vi "Get Full Decay Fit & Residual Plots (1-Exp Fit).vi"(4 "Laser Period":dbl[unit], 6 "Fit Options":T2={"Show Fit Residuals"=TRUE, "Fit Model"=enum."1-Exponential", "Residual Type"=enum."Standard", "Max Decay Percentile"=0.0, "Min Decay Percentile"=0.0, "Show Full Decay"=TRUE, "Weights"=enum."Unweighted", "Fitting Method"=enum."Least Square", "Compute Parameter Uncertainties"=TRUE, "Periodic Boundaries"=TRUE, "Model Calculation"=enum."Simulation", "Period"=1.2500000000000001e-08, "Termination Criteria"={"Max Iterations"=1000, "Max Function Calls"=0, "Max Time"=1000.0, "Function Tolerance"=1e-06, "Parameter Tolerance"=1e-06, "Gradient Tolerance"=0.0, "Min Lambda"=1e-06, "Max Lambda"=1e-06, "Initial Tick Count"=0}, "Offset Resolution"=1.2500000000000001e-08, "Use Local IRF"=TRUE, "Fitting Algorithm"=enum."Levenberg-Marquardt", "Show Confidence Interval "=TRUE, "Confidence Level"=95.0} {"Confidence Level" min=0.0 max=100.0; "Offset Resolution" min=0.0; "Period" min=0.0; "Min Decay Percentile" min=0.0 max=1.0; "Max Decay Percentile" min=0.0 max=100.0}, 8 "Error In":errorcluster, 9 "Best Fit Parameters (All)":dbl[](array[numeric]), 10 "IRF":cluster{"t Array":dbl[], "IRF Array":dbl[]}, 11 "Full Decay":cluster{"t Array":dbl[], "Y Array":dbl[]}) -> (0 "Error Out":errorcluster, 3 "Fit Plots":T1)   [LabVIEW 2021, in "Fits.lvlib"]
uses:
  Fits.lvlib
  Decay Fit Options v4.ctl
  Decay Convolution/Decay Model.ctl
  Residual Type.ctl
  Fit Weights Type v2.ctl
  Non-linear Fitting Method v2.ctl
  Fit Calculation Method.ctl
  Non-linear Fitting Algorithm.ctl
  Fit Plots.ctl
  Decay Convolution/Fit Control Data.ctl
  Graphs/XY Graph/XY Graph Plot Data.ctl
  Graphs/XY Graph/XY Graph Add-Ons.lvlib
panel:
  out "XY Graph":cluster{"t Array":dbl[], "f(X,a)":dbl[]}[](graph)
  # "see the License on the block diagram (Ctrl+E or Window:Show Block Diagram)"
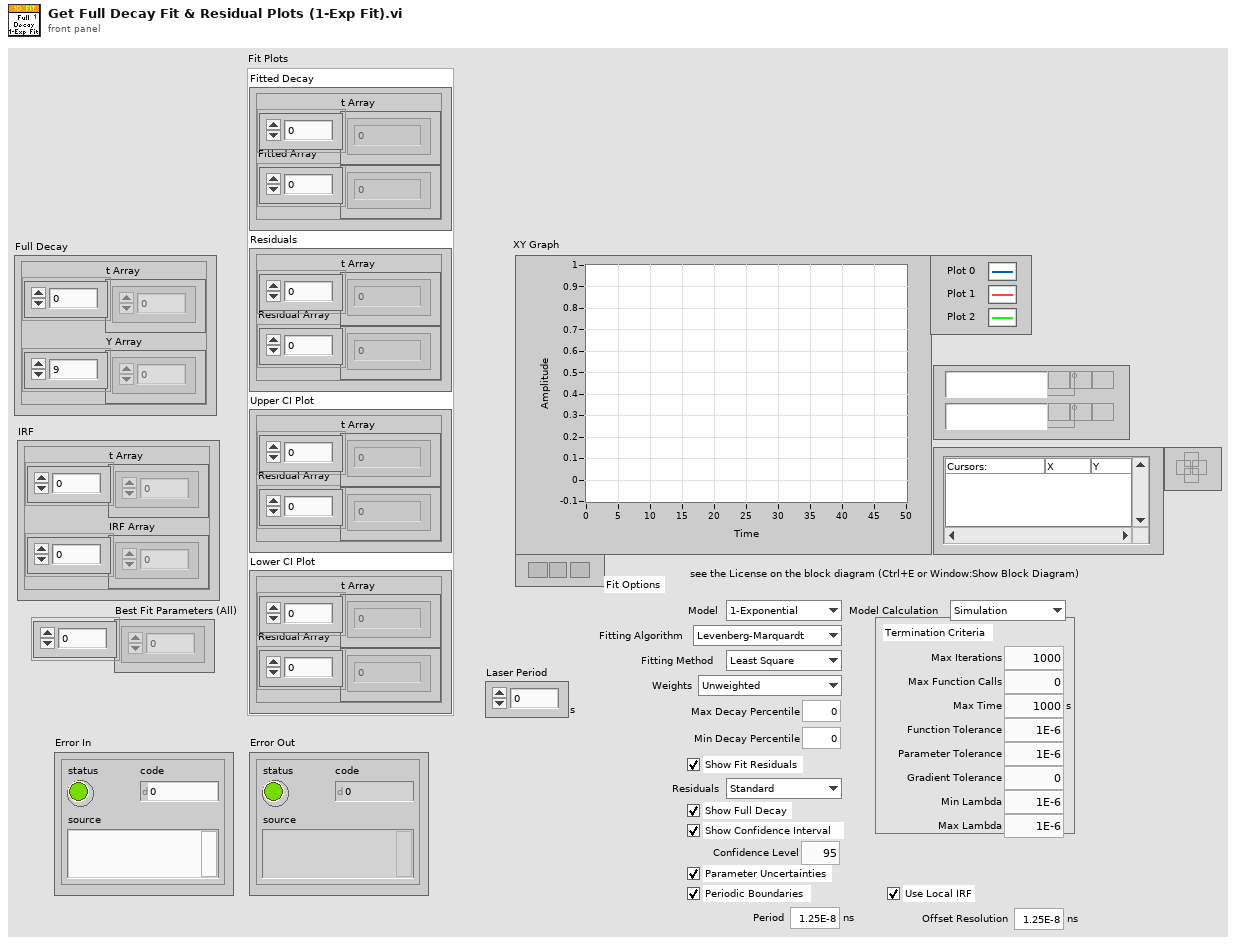
[diagram p1: front panel]
types:
  T1 = typedef "Fits.lvlib/Fit Plots.ctl" = cluster{"Fitted Decay":cluster{"t Array":dbl[], "Fitted Array":dbl[]}, "Residuals":cluster{"t Array":dbl[], "Residual Array":dbl[]}, "Upper CI Plot":cluster{"t Array":dbl[], "Residual Array":dbl[]}, "Lower CI Plot":cluster{"t Array":dbl[], "Residual Array":dbl[]}}
  T2 = typedef "Fits.lvlib/Decay Fit Options v4.ctl" = cluster{"Show Fit Residuals":bool, "Fit Model":T3, "Residual Type":T4, "Max Decay Percentile":dbl, "Min Decay Percentile":dbl, "Show Full Decay":bool, "Weights":T5, "Fitting Method":T6, "Compute Parameter Uncertainties":bool, "Periodic Boundaries":bool, "Model Calculation":T7, "Period":dbl[unit], "Termination Criteria":cluster{"Max Iterations":i32, "Max Function Calls":i32, "Max Time":dbl[unit], "Function Tolerance":dbl, "Parameter Tolerance":dbl, "Gradient Tolerance":dbl, "Min Lambda":dbl, "Max Lambda":dbl, "Initial Tick Count":u32}, "Offset Resolution":dbl[unit], "Use Local IRF":bool, "Fitting Algorithm":T8, "Show Confidence Interval ":bool, "Confidence Level":dbl}
  T3 = typedef "Fits.lvlib/Decay Model.ctl" = enum16{"1-Exponential", "2-Exponentials"}
  T4 = typedef "Fits.lvlib/Residual Type.ctl" = enum16{"Standard", "Normalized", "Reduced"}
  T5 = typedef "Fits.lvlib/Fit Weights Type v2.ctl" = enum16{"Unweighted", "1/Variance (Neyman)", "1/Variance (Pearson)", "Best of All"}
  T6 = typedef "Fits.lvlib/Non-linear Fitting Method v2.ctl" = enum16{"Least Square", "Least Absolute Residual", "Bisquare", "MLE", "-", "Best of All"}
  T7 = typedef "Fits.lvlib/Fit Calculation Method.ctl" = enum16{"Simulation", "Convolution", "Integration"}
  T8 = typedef "Fits.lvlib/Non-linear Fitting Algorithm.ctl" = enum16{"Levenberg-Marquardt", "Trust-Region Dogleg"}
  T9 = typedef "Fits.lvlib/Fit Control Data.ctl" = cluster{"IRF":T10, "Laser Period":dbl, "SYNC Period":dbl}
  T10 = typedef "XY Graph Add-Ons.lvlib/XY Graph Plot Data.ctl" = cluster{"X Array":dbl[], "Y Array":dbl[]}
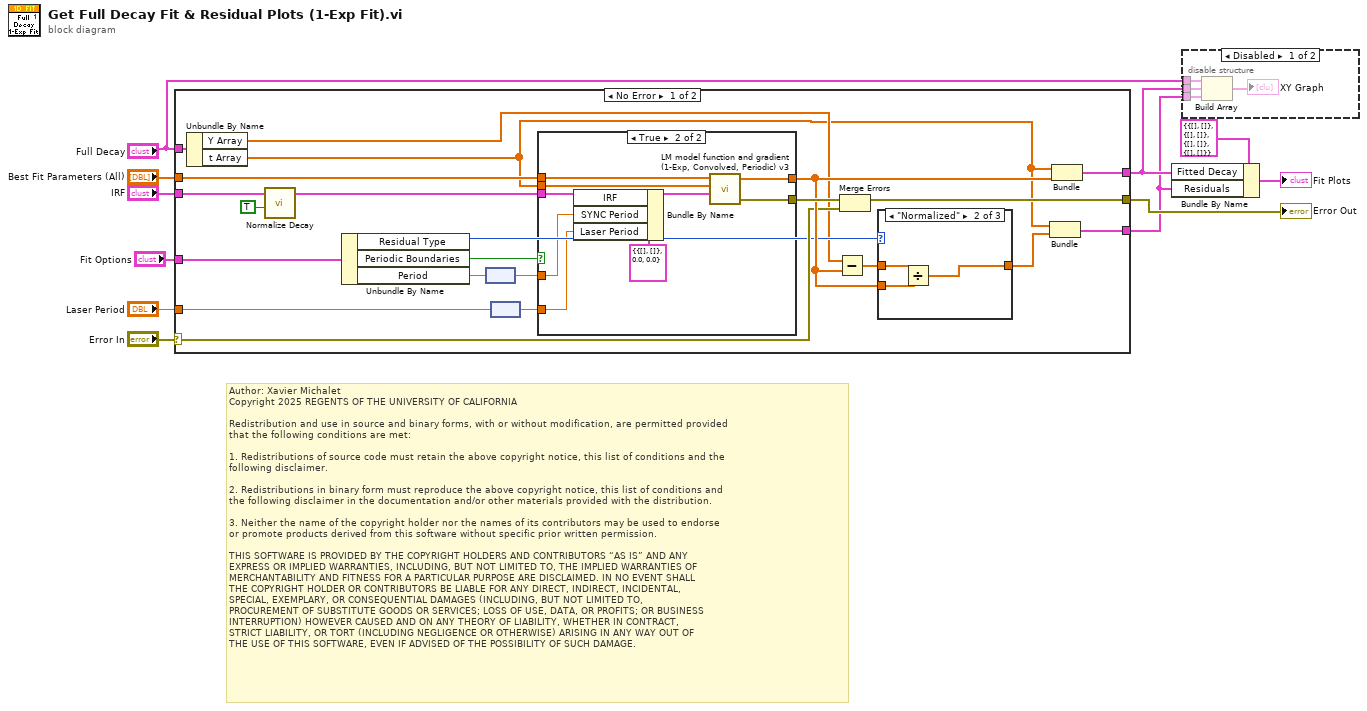
[diagram p0: block diagram]
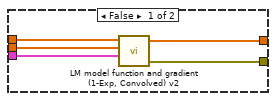
[diagram p3: hidden frame]
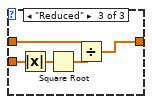
[diagram p5: hidden frame]
diagram:
  # "Author: Xavier Michalet\nCopyright 2025 REGENTS OF THE UNIVERSITY OF CALIFORNIA\n\nRedistribution and use in source and binary forms, with or without modification, are permitted provided\nthat the following conditions are met:\n\n1. Redistributions of source code must retain the above copyright notice, this list of conditions and the\nfollowing disclaimer.\n\n2. Redistributions in binary form must reproduce the above copyright notice, this list of conditions and\nthe following disclaimer in the documentation and/or other materials provided with the distribution.\n\n3. Neither the name of the copyright holder nor the names of its contributors may be used to endorse \nor promote products derived from this software without specific prior written permission.\n\nTHIS SOFTWARE IS PROVIDED BY THE COPYRIGHT HOLDERS AND CONTRIBUTORS “AS IS” AND ANY \nEXPRESS OR IMPLIED WARRANTIES, INCLUDING, BUT NOT LIMITED TO, THE IMPLIED WARRANTIES OF\nMERCHANTABILITY AND FITNESS FOR A PARTICULAR PURPOSE ARE DISCLAIMED. IN NO EVENT SHALL\nTHE COPYRIGHT HOLDER OR CONTRIBUTORS BE LIABLE FOR ANY DIRECT, INDIRECT, INCIDENTAL, \nSPECIAL, EXEMPLARY, OR CONSEQUENTIAL DAMAGES (INCLUDING, BUT NOT LIMITED TO, \nPROCUREMENT OF SUBSTITUTE GOODS OR SERVICES; LOSS OF USE, DATA, OR PROFITS; OR BUSINESS\nINTERRUPTION) HOWEVER CAUSED AND ON ANY THEORY OF LIABILITY, WHETHER IN CONTRACT, \nSTRICT LIABILITY, OR TORT (INCLUDING NEGLIGENCE OR OTHERWISE) ARISING IN ANY WAY OUT OF\nTHE USE OF THIS SOFTWARE, EVEN IF ADVISED OF THE POSSIBILITY OF SUCH DAMAGE."
  n1 = case shown="No Error" "Error In" {
    selector: "Error In" -> [w23 w57]
    tunnel: "IRF" -> [w16 _]
    tunnel: "Best Fit Parameters (All)" -> [w25 _]
    tunnel: [w33 _] -> w2
    tunnel: "Fit Options" -> [w32 _]
    tunnel: [w24 w57] -> w8
    tunnel: [w29 _] -> w1
    tunnel: "Full Decay" -> [w27 _]
    tunnel: "Laser Period" -> [w22 _]
    frame No Error {
      n2 = Unbundle By Name(w27) -> ("Y Array"=w13:dbl[], "t Array"=w12:dbl[])
      n3 = call "Normalize Decay.vi"("IRF (F)"=TRUE, "Decay"=w16) -> ("Normalized Decay"=w15:cluster{"t Array":dbl[], "Y Array":dbl[]})  [unwired: 7 in, 2 out]
      n4 = Unbundle By Name(w32) -> ("Residual Type"=w21:T4, "Periodic Boundaries"=w20:bool, "Period"=w19:dbl[unit])
      n5 = node(w19) -> (w18:dbl)
      n6 = node(w22) -> (w17:dbl)
      n7 = case shown="True" w20 {
        tunnel: [w38 w44] -> w31
        tunnel: [w37 w45] -> w28
        tunnel: w15 -> [w36 w41]
        tunnel: w12 -> [w35 w47]
        tunnel: w25 -> [w34 w46]
        tunnel: w17 -> [_ w40]
        tunnel: w18 -> [_ w39]
        frame False {
          n8 = call "LM model function and gradient (1-Exp, Convolved) v2.vi"("data"=w36, "X"=w35, "a"=w34) -> ("error out"=w38:errorcluster, "f(X,a)"=w37:dbl[])  [unwired: 1 in, 1 out]
        }
        frame True {
          n9 = Bundle By Name(cluster=T9 {"IRF"={"X Array"=[], "Y Array"=[]}, "Laser Period"=0.0, "SYNC Period"=0.0} ("Fit Control Data"), "IRF"=w41, "SYNC Period"=w39, "Laser Period"=w40) -> (w43:T9)
          n10 = call "LM model function and gradient (1-Exp, Convolved, Periodic) v3.vi"("data"=w43, "X"=w47, "a"=w46) -> ("error out"=w44:errorcluster, "f(X,a)"=w45:dbl[])  [unwired: 1 in, 1 out]
        }
      }
      n11 = Subtract(x=w13, y=w28) -> (x-y=w26:dbl[])
      n12 = Merge Errors(w31, w23) -> (w24:errorcluster)
      n13 = case shown="\"Normalized\"" w21 {
        tunnel: w26 -> [w48 w51 w56]
        tunnel: [w48 w49 w54] -> w30
        tunnel: w28 -> [_ w50 w55]
        frame "Standard", Default {
        }
        frame "Normalized" {
          n14 = Divide(x=w51, y=w50) -> (x/y=w49:dbl[])
        }
        frame "Reduced" {
          n15 = Absolute Value(x=w55) -> (abs(x)=w53:dbl[])
          n16 = Square Root(x=w53) -> (sqrt(x)=w52:dbl[])
          n17 = Divide(x=w56, y=w52) -> (x/y=w54:dbl[])
        }
      }
      n18 = Bundle("t Array"=w12, w30) -> (w29:cluster{"t Array":dbl[], dbl[]})  [unwired: 1 in]
      n19 = Bundle("t Array"=w12, "f(X,a)"=w28) -> (w33:cluster{"t Array":dbl[], "f(X,a)":dbl[]})  [unwired: 1 in]
    }
    frame Error {
    }
  }
  "Error Out" <- w8
  n20 = Bundle By Name(cluster=T1 {"Fitted Decay"={"t Array"=[], "Fitted Array"=[]}, "Residuals"={"t Array"=[], "Residual Array"=[]}, "Upper CI Plot"={"t Array"=[], "Residual Array"=[]}, "Lower CI Plot"={"t Array"=[], "Residual Array"=[]}} ("Fit Plots"), "Fitted Decay"=w2, "Residuals"=w1) -> (→"Fit Plots":T1)
  n21 = disable-structure shown="Disabled" {
    disable-tunnel: "Full Decay" -> [w61 _]
    disable-tunnel: w2 -> [w60 _]
    disable-tunnel: w1 -> [w59 _]
    frame Disabled {
      n22 = Build Array(w61, w60, w59) -> (→"XY Graph":cluster{"t Array":dbl[], "f(X,a)":dbl[]}[])
    }
    frame Enabled {
    }
  }
